vi "Error Analysis (SubVI).vi"(10 "Measured Wave":dbl[](array[numeric]), 11 "Reference Wave":dbl[](array[numeric])) -> (1 "RMSE":dbl=2.4180691084086257, 2 "Sum of LSE":dbl=2689.6467779984355, 3 "Absolute Error Plot":dbl[](graph)=[4.289049738671714, 4.2138371310211795, 4.103388077383556, 3.9557882936772444, 3.7744944440454375, 3.5637991245828715, 3.325165549201813, 3.0556431592000735, 2.747501359979559, 2.391807083165652, 1.9784739377349325, 1.5039241579374831, 0.9701306984907703, 0.38686354967651937, 0.23531054496175585, 0.8722819147657361, 1.5167294133948275, 2.1446984801556894, 2.7490594924048253, 3.3145084508691838, 3.8407367361648, 4.320600958075026, 4.761954937878649, 5.157193011969696, 5.5241666956922515, 5.853474706908621, 6.152548799696028, 6.421158729727381, 6.661734206282674, 6.866711522296789, 7.037711282981263, 7.180448615219575, 7.290650503352808, 7.369011897235183, 7.42170117406058, 7.450728311224111, 7.459038432242039, 7.455147611276573, 7.438327983423825, 7.412099147766909, 7.386290028587773, 7.363607633300688, 7.343621376843814, 7.323187312117824, 7.304654096610676, 7.2840335425818665, 7.26691756542067, 7.243021719379527, 7.210728568123258, 7.174377402498038, 7.126518457528249, 7.0659346275323, 6.995627651375585, 6.918687913579575, 6.823385811242531, 6.713125533684206, 6.591490124117371, 6.452332041641085, 6.294680341948819, 6.117784903094133, 5.921068819124059, 5.704217841568465, 5.46713222087692, 5.214924057181264, 4.943097496753879, 4.657591358170976, 4.3595468765546315, 4.050487215329895, 3.732267908213899, 3.4118898040466803, 3.09149496651294, 2.7682251259015374, 2.4442631384753923, 2.1266455027493407, 1.8173952683299888, 1.5081971849291307, 1.2107137346529697, 0.9263061414514766, 0.6462590013538829, 0.38168460665322357, 0.12342742378517357, 0.11266504066057337, 0.34102046596990476, 0.5511619466525701, 0.7478026064031269, 0.9258483683155418, 1.0903088590466297, 1.2414368554259596, 1.379592725956897, 1.5001542811730104, 1.6137466743299456, 1.7058768345057018, 1.7921168141884607, 1.8629663155815734, 1.9238979278515842, 1.9753104279662352, 2.0074817054045866, 2.035567099494088, 2.0446889423278236, 2.0498426763708295, 2.035940002121606, 2.017943312900087, 1.985587925305424, 1.9437449874902768, 1.8921891814393632, 1.83064101687836, 1.7588549130365294, 1.6816158263083736, 1.5935987437841845, 1.4993658011122761, 1.403730015535075, 1.2963413641320898, 1.1918685858719016, 1.0799070747881387, 0.9704368988708723, 0.8632288367318921, 0.7581209749469835, 0.6603875726446589, 0.5714746311608039, 0.4877215035957505, 0.4223531894323287, 0.3693190044621275, 0.32950729565781955, 0.31073535718681455, 0.31059087169555966, 0.3176699622343264, 0.3372147769037497, 0.3605515749231927, 0.38498211825261563, 0.4219377782373144, 0.5045529219553231, 0.635013004115919, 0.7975741337654583, 0.988726990753527, 1.1880575997474807, 1.3792575190600402, 1.5561309417897604, 1.7221362978888948, 1.886669796981849, 2.0527872233157893, 2.2158264383811, 2.3575185510466383, 2.4591004229509963, 2.499478225081589, 2.4833564041944243, 2.3973121836027502, 2.2609604838430144, 2.089255215767679, 1.9040892683277733, 1.722395007140598, 1.5566561980999936, 1.4106207525200603, 1.2925936568388465, 1.1935999302400688, 1.116300820288835, 1.0413262955028344, 0.9745649429068735, 0.9004074662269872, 0.8220034784031967, 0.7467070721408291, 0.6702520204882418, 0.6012632055410094, 0.5530298486376211, 0.5303447728200368, 0.5301737099626322, 0.5550088811435856, 0.6060100657705476, 0.6723032154125406, 0.7514787687751436, 0.8401415788437063, 0.9297378305829795, 1.0167403673877047, 1.0927392385837393, 1.15961873310048, 1.2093161992476809, 1.2492149383987154, 1.2770267720582211, 1.2961717527753152, 1.310831771963251, 1.3160909393141225, 1.3226144013779972, 1.3262785434655129, 1.3278907929516706, 1.3181371263016075, 1.3124374890454575, 1.2964420299482668, 1.275703690187754, 1.2509464218850397, 1.2178763325383883, 1.187130889425596, 1.1545035045550804, 1.125756822387217, 1.0968485997102704, 1.0735172609688988, 1.0566918617729257, 1.0421700155239364, 1.0355249974848064, 1.0371504141930146, 1.0372135098254347, 1.0404712927664335, 1.0416818575658056, 1.0453291637060858, 1.050942965806854, 1.0530525961581958, 1.061186568778652, 1.0649637732128028, 1.0691389264733218, 1.0684649530554822, 1.072784269812196, 1.0769827699961425, 1.080898056084365, 1.084410797756476, 1.0823987857897635, 1.084553681121136, 1.08074709062209, 1.0706642553909447, 1.0641243908552127, 1.0510348418928572, 1.0413452561329066, 1.025276427612873, 1.0129083003977755, 0.994591946858236, 0.9807664798706384, 0.9667302039540644, 0.9579610858320464, 0.9447963810696223, 0.9375700275753402, 0.9265211729245095, 0.9218858140498583, 0.913805344639961, 0.9072808868679232, 0.9024022840798409, 0.8991193459411022, 0.8924708549319931, 0.892355823781763, 0.8938082882403577, 0.8917227983570513, 0.8960834436618299, 0.8967809019003994, 0.903612591926148, 0.9065117055777421, 0.9102727101828378, 0.9146430552498614, 0.9194606543773745, 0.924470937951078, 0.9244643328444369, 0.9293221892577606, 0.9288796032349396, 0.9280171137336595, 0.931706620907697, 0.9299199742170359, 0.9326748828700175, 0.9314892708173446, 0.9314271778886862, 0.9315531048271524, 0.9308405774162907, 0.9303553578187831, 0.9296639970966467, 0.9282881570837418, 0.9272047014261986, 0.9255288820807195, 0.9247397643768593, 0.9228634001907778, 0.9220186678681586, 0.921234227868581, 0.9205401244041482, 0.9200136046758942, 0.9196876047482192, 0.9195507795024014, 0.919730627682732, 0.9200815288946558, 0.9207340590589794, 0.9210914631827123, 0.921058529401769, 0.9212246812284803, 0.920951982367427, 0.9206955432765227, 0.9195034935565474, 0.918742295855516, 0.916962911162102, 0.9150803267154544, 0.9131023848105997, 0.910992403096003, 0.9082606679045568, 0.9048270460636445, 0.9012497967441604, 0.8969508494659735, 0.8924446091810978, 0.8877463300487847, 0.8818262620766149, 0.876201121909375, 0.8698424597064829, 0.8633596772598011, 0.8567710654357867, 0.8495494935119865, 0.8428511997714025, 0.8356037249913086, 0.8289178046055525, 0.8218584044144777, 0.8148988588566297, 0.8081496631268834, 0.8010379607641269, 0.7946736650544466, 0.788074725549464, 0.7817586006177635, 0.7756964060047551, 0.7694501680588388, 0.7635812025456303, 0.7580127212384866, 0.7528044213587748, 0.7479693239237761, 0.7435194934642411, 0.7390117619012813, 0.7348645793584367, 0.7311326243249425, 0.72782366367084, 0.7243985194137252, 0.7213625913940405, 0.7187658340316219, 0.716019636283221, 0.7142172371098354, 0.7122675139465287, 0.7107154086867453, 0.7090130531506844, 0.7082486546469084, 0.707326080970013, 0.7067853073340231, 0.7065735626125615, 0.7062742354131757, 0.7067864792482652, 0.7071914547047982, 0.7079319439735201, 0.7089497246362129, 0.7098229476919755, 0.71099154026858, 0.712440366968579, 0.7141535173662419, 0.7156143722975443, 0.7173514486730923, 0.7193011451179814, 0.7214451429726338, 0.7233562584875912, 0.7253780930013178, 0.7275828678506358, 0.7299510772687441, 0.7319173460086432, 0.7340078384581332, 0.7361572395611233, 0.7383461639657725, 0.7400554627485079, 0.7418120802745065, 0.7435060324815836, 0.7447109139855641, 0.7458177711318896, 0.7473556051666961, 0.7478541181528513, 0.7487064561677315, 0.7489439288488455, 0.7490071953643422, 0.7489752016972133, 0.7487448083854318, 0.7478512710540883, 0.7467851864680597, 0.7454925361668288, 0.7440120520370854, 0.7423379243359349, 0.7399198313902744, 0.7373460663559896, 0.7345231287170506, 0.7314961675403424, 0.7283116648647763, 0.7243801140420203, 0.720750672385563, 0.7159738294696112, 0.7114640704779518, 0.7068202895066236, 0.7015053413282999, 0.6960291188055194, 0.6904027483624589, 0.6846843320491658, 0.6783415834720188, 0.6718891126069124, 0.6658426048698303, 0.658718772076547, 0.6520810755220694, 0.6449023440083295, 0.6382020419014651, 0.6310004326526624, 0.6233185154670338, 0.6162237353973126, 0.6091925897296022, 0.6017478857754242, 0.5944128955289756, 0.5867112848924663, 0.5796670422746217, 0.5728044068482987, 0.5651935722329497, 0.5582675129830719, 0.5515965663978051, 0.5447510357432108, 0.5381637944901527, 0.5324506466445484, 0.5260440563369784, 0.5200592868668181, 0.5149739094476473, 0.5097650689276563, 0.5050467518451427, 0.5007950776487675, 0.497031347416808, 0.4932304424953884, 0.4900038789800547, 0.4873251104295946, 0.4852125885681957, 0.48318394981608037, 0.4817559806132934, 0.4814445861053045, 0.4807647622265563, 0.48127634668577457, 0.4824008959618169, 0.48369632054394884, 0.4857195442199469, 0.48838916672107047, 0.4918058845029236, 0.49538628252932426, 0.5002290369537832, 0.5052487131628141, 0.5110419745372425, 0.5175671618589277, 0.5242816303206297, 0.532279089189629, 0.5405149646511518, 0.5494895198712939, 0.5592020998968081, 0.5691511541444356, 0.5803342608487156, 0.5917481533172477, 0.6038887478400952, 0.6167511730989759, 0.6298298009210015, 0.6441640537051754, 0.6586553354708542, 0.6738417186262637, 0.6897606522530353, 0.7063116726813874, 0.7230768883856626, 0.7410007868576045, 0.7585291911568248, 0.7772709901143813, 0.7967411441151455, 0.8174575152789672, 0.8391830601259542, 0.8668633833548967, 0.9071342736733925, 0.9861450453187075, 1.1639432032863795, 1.5172339554602772, 2.0763219680864395, 2.7605542080817997, 3.360144147510823, 3.6202697046473276], 4 "Max. Absolute Error":dbl=7.459038432242039)   [LabVIEW 2017]
uses:
  <vilib>/Analysis/NI_AALPro.lvlib
  <vilib>/Analysis/5stat.llb/RMS (DBL).vi
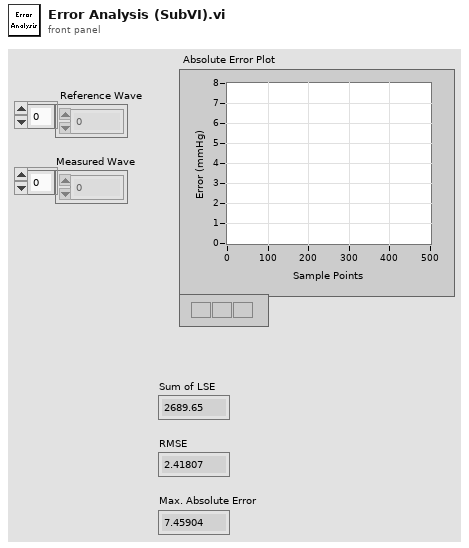
[diagram p1: front panel]
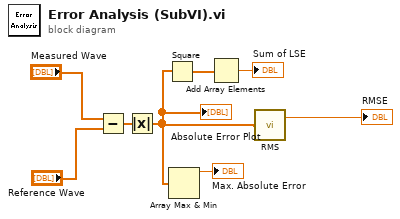
[diagram p0: block diagram]
diagram:
  n1 = Subtract(x="Measured Wave", y="Reference Wave") -> (x-y=w1:dbl[])
  n2 = Absolute Value(x=w1) -> (abs(x)=w7:dbl[])
  "Absolute Error Plot" <- w7
  n3 = Square(x=w7) -> (x^2=w2:dbl[])
  n4 = Array Max & Min(array=w7) -> (max value=→"Max. Absolute Error":dbl)  [unwired: 3 out]
  n5 = Add Array Elements(numeric array=w2) -> (sum=→"Sum of LSE":dbl)
  n6 = call-poly <vilib>:"RMS.vi"("X"=w7) -> ("rms value"=→"RMSE":dbl)  [unwired: 1 out]
